vi "TDMS Copy File Except Specified Groups.vi"(7 "Groups Names":string[](array[string]), 8 "error in (no error)":errorcluster, 10 "TDMS Destination In":refnum<k34>, 11 "TDMS Source In":refnum<k34>) -> (0 "error out":errorcluster, 2 "TDMS Destination Out":refnum<k34>, 3 "TDMS Source Out":refnum<k34>)   [LabVIEW 2011]
doc: "Copies all the channels and properties from the source file to the destination file."
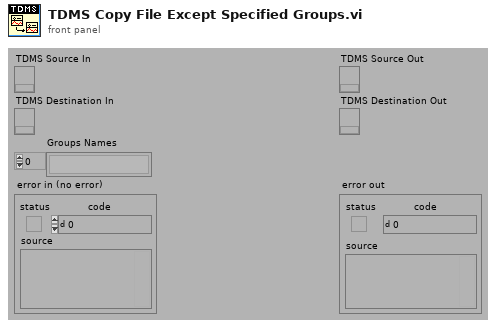
[diagram p1: front panel]
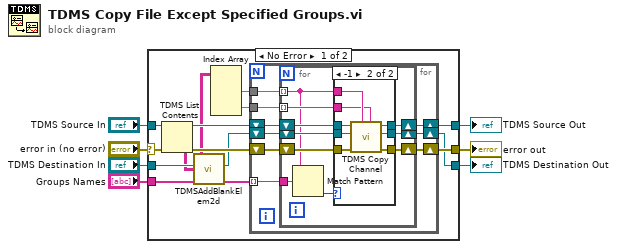
[diagram p0: block diagram]
diagram:
  n1 = case shown="No Error" "error in (no error)" {
    selector: "error in (no error)" -> [w12 w53]
    tunnel: "TDMS Destination In" -> [w11 w51]
    tunnel: "TDMS Source In" -> [w20 w52]
    tunnel: [w17 w52] -> w5
    tunnel: [w10 w51] -> w4
    tunnel: [w13 w53] -> w3
    tunnel: "Groups Names" -> [w9 _]
    frame No Error {
      n2 = TDMS List Contents(4:w12, 7:w20) -> (0:w19:errorcluster, 1:w8:string[][], 3:w18:refnum<k34>)  [unwired: 2 out]
      n3 = call <vilib>:"TDMSAddBlankElem2d.vi"("input 2d string array"=w8) -> ("output 2d string array with the first column blank"=w16:string[][])
      n4 = Index Array(array=w16) -> (element #1=w15:string[], element #2=w14:string[])  [unwired: 4 in]
      n5 = for {
        tunnel: w15 -> [w26]
        tunnel: w14 -> [w25]
        shift-right: [w27] -> w17
        shift-left: w18 -> [w28]
        shift-right: [w22] -> w10
        shift-left: w11 -> [w23]
        shift-right: [w24] -> w13
        shift-left: w19 -> [w29]
        tunnel: w9 -> [w21] mode=indexing
        n6 = for {
          shift-right: [w38] -> w24
          shift-left: w29 -> [w35]
          shift-right: [w37] -> w22
          shift-left: w23 -> [w39]
          shift-right: [w36] -> w27
          shift-left: w28 -> [w34]
          tunnel: w26 -> [w31] mode=indexing
          tunnel: w25 -> [w33] mode=indexing
          tunnel: w21 -> [w32]
          n7 = Match Pattern(string=w31, regular expression=w32) -> (offset past match=w30:i32)  [unwired: 4 out]
          n8 = case shown="-1" w30 {
            tunnel: w39 -> [w41 w50]
            tunnel: [w42 w49] -> w38
            tunnel: [w41 w48] -> w37
            tunnel: [w40 w47] -> w36
            tunnel: w35 -> [w42 w46]
            tunnel: w34 -> [w40 w45]
            tunnel: w31 -> [_ w44]
            tunnel: w33 -> [_ w43]
            frame Default {
            }
            frame -1 {
              n9 = call "TDMS Copy Channel.vi"("channel name"=w43, "group name"=w44, "error in"=w46, "tdms dest in"=w50, "tdms source in"=w45) -> ("error out"=w49:errorcluster, "tdms dest out"=w48:refnum<k34>, "tdms source out"=w47:refnum<k34>)  [unwired: 4 out]
            }
          }
        }
      }
    }
    frame Error {
    }
  }
  "TDMS Source Out" <- w5
  "TDMS Destination Out" <- w4
  "error out" <- w3
